vi "Read string to array.vi"(4 "String":string) -> (0 "size(s)":i32, 1 "Array":i32[](array[numeric]), 2 "caracter":string)   [LabVIEW 2013]
panel:
  out "Actual":string
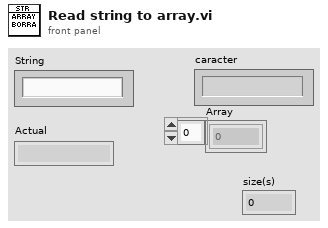
[diagram p1: front panel]
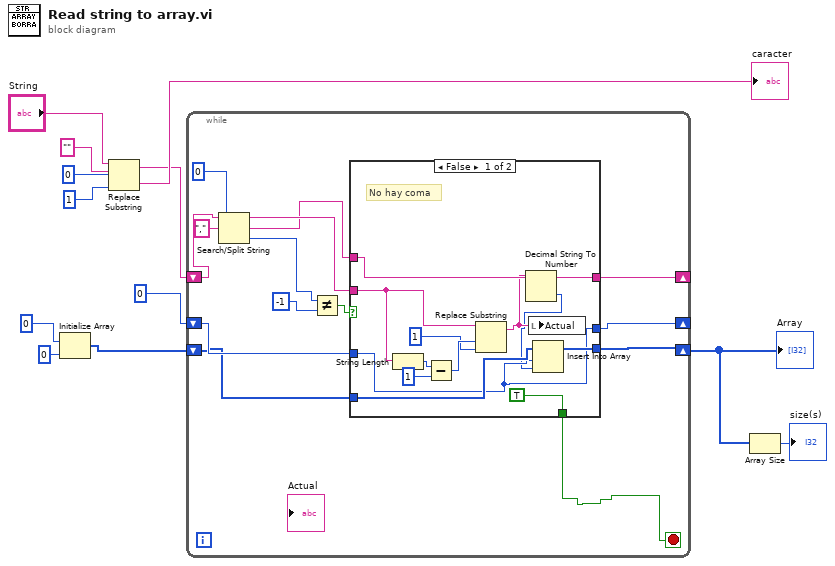
[diagram p0: block diagram]
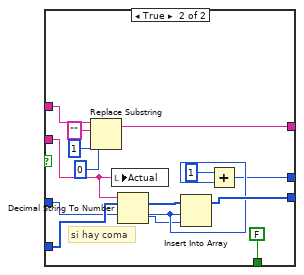
[diagram p2: hidden frame]
diagram:
  n1 = Initialize Array(0, 0 ("dimension size")) -> (w1:i32[])
  n2 = Replace Substring(2:1 ("length (len. of substring)"), 3:0 ("offset (0)"), 4:"" ("substring (\"\")"), 5:"String") -> (0:→"caracter":string, 1:w7:string)
  n3 = while {
    shift-right: [w18] -> _
    shift-left: w7 -> [w21]
    shift-right: [w15] -> w4
    shift-left: w1 -> [w16]
    shift-right: [w14] -> _
    shift-left: 0 -> [w17]
    stop <- w13 stop-if-true
    n4 = Search/Split String(string=w21, search string/char (-)=",", offset (0)=0) -> (substring before match=w22:string, match + rest of string=w19:string, offset of match=w24:i32)
    n5 = Not Equal?(x=w24, y=-1) -> (x != y?=w20:bool)
    n6 = case shown="False" w20 {
      tunnel: w22 -> [w38 w40]
      tunnel: [TRUE FALSE] -> w13
      tunnel: w19 -> [w32 w50]
      tunnel: [w32 w46] -> w18
      tunnel: w17 -> [w29 w43]
      tunnel: w16 -> [w31 w45]
      tunnel: [w30 w44] -> w15
      tunnel: [w29 w41] -> w14
      frame False {
        # "No hay coma"
        n7 = String Length(string=w38) -> (length=w37:i32)
        n8 = Subtract(x=w37, y=1) -> (x-y=w35:i32)
        n9 = Replace Substring(2:1 ("length (len. of substring)"), 3:w35, 5:w38) -> (1:w28:string)  [unwired: 1 in, 1 out]
        n10 = Decimal String To Number(string=w28) -> (number=w27:i32)  [unwired: 2 in, 1 out]
        n11 = local write "Actual"(w28) -> ()
        n12 = Insert Into Array(array=w31, index=w29, new element=w27) -> (w30:i32[])
      }
      frame True {
        # "si hay coma"
        n13 = Replace Substring(2:1 ("length (len. of substring)"), 3:0 ("offset (0)"), 4:"" ("substring (\"\")"), 5:w50) -> (1:w46:string)  [unwired: 1 out]
        n14 = local write "Actual"(w40) -> ()
        n15 = Decimal String To Number(string=w40) -> (number=w39:i32)  [unwired: 2 in, 1 out]
        n16 = Insert Into Array(array=w45, index=w43, new element=w39) -> (w44:i32[])
        n17 = Add(x=1, y=w43) -> (x+y=w41:i32)
      }
    }
  }
  "Array" <- w4
  n18 = Array Size(array=w4) -> (size(s)=→"size(s)":i32)
